vi "pwn_v1.vi"() -> ()   [LabVIEW 2017]
panel:
  out "Waveform Chart":i32(graph)
  in  "Slide":dbl(slide) scale=0.0..190.0
  in  "stop":bool
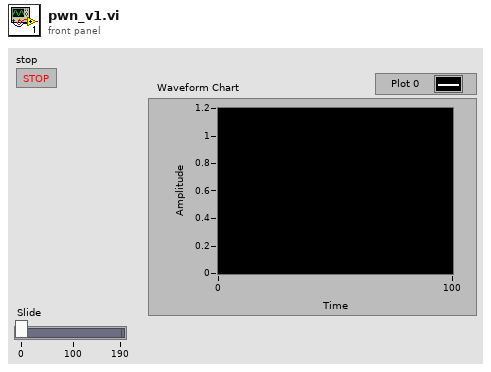
[diagram p1: front panel]
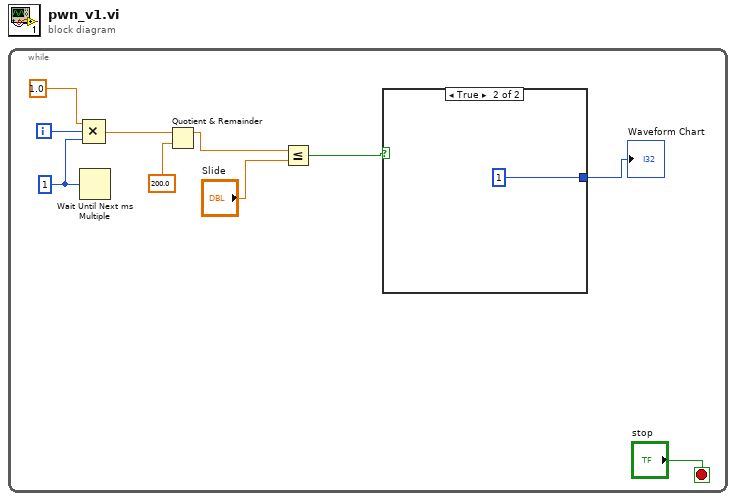
[diagram p0: block diagram]
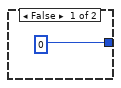
[diagram p2: hidden frame]
diagram:
  n1 = while {
    i -> [w8]
    stop <- "stop" stop-if-true
    w9 = u32 1 ("millisecond multiple")
    n2 = Wait Until Next ms Multiple(millisecond multiple=w9) -> ()  [unwired: 1 out]
    n3 = Compound Arithmetic op=MULTIPLY(1.0, w8, w9) -> (w5:dbl)
    n4 = Quotient & Remainder(x=w5, y=200.0) -> (x-y*floor(x/y)=w4:dbl)  [unwired: 1 out]
    n5 = Less Or Equal?(x=w4, y="Slide") -> (x <= y?=w3:bool)
    n6 = case shown="True" w3 {
      tunnel: [0 1] -> w1
      frame False {
      }
      frame True {
      }
    }
    "Waveform Chart" <- w1
  }
